vi "Laboratory_practice10.vi"() -> ()   [LabVIEW 2021]
panel:
  out "volts":dbl
  in  "Wait time(ms)":dbl
  in  "number of samples":i32=100
  in  "rate":dbl=5000.0
  out "Waveform Graph":dynamicdata(graph)
  in  "Traditional DAQ Channel":tag
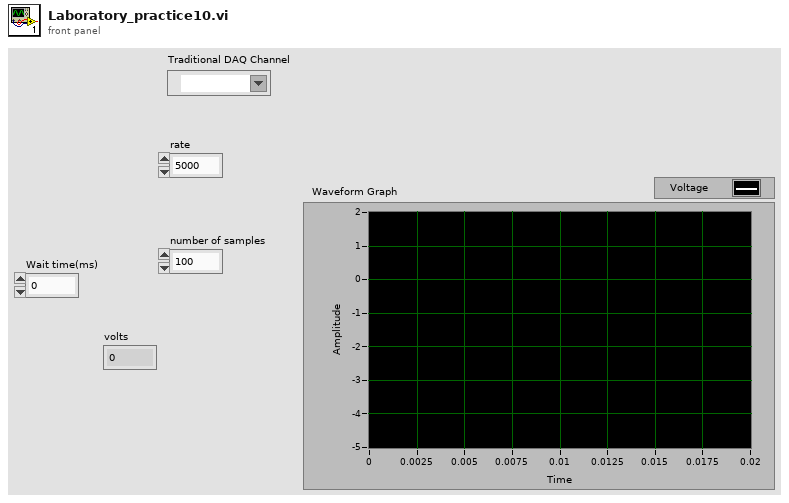
[diagram p1: front panel]
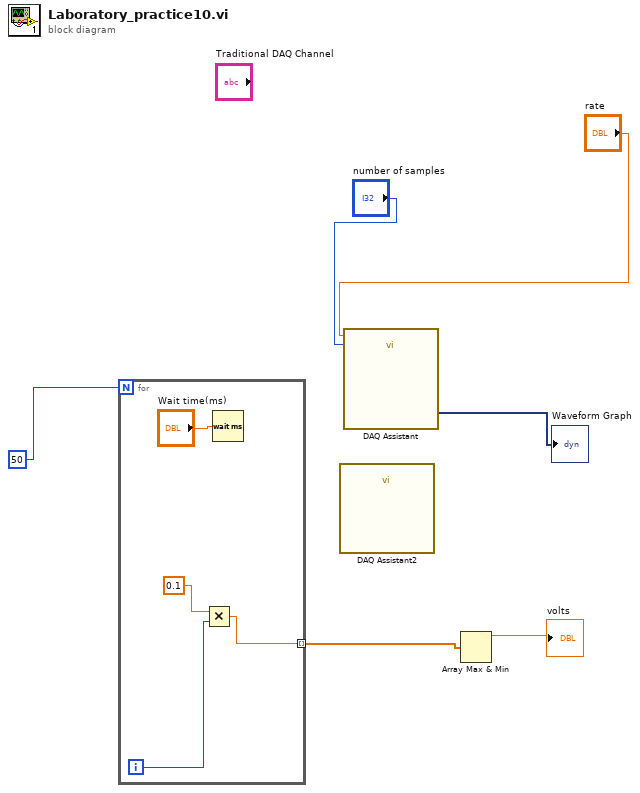
[diagram p0: block diagram]
diagram:
  n1 = for {
    N: 50 -> [_]
    tunnel: [w7] -> w2 mode=indexing
    i -> [w8]
    n2 = Multiply(x=0.1, y=w8) -> (x*y=w7:dbl)
    n3 = Wait (ms)(milliseconds to wait="Wait time(ms)") -> ()  [unwired: 1 out]
  }
  n4 = call "DAQ Assistant2"() -> ()  [unwired: 18 in, 2 out]
  n5 = call "DAQ Assistant"("rate"="rate", "number of samples"="number of samples") -> ("data"=→"Waveform Graph":dynamicdata)  [unwired: 15 in, 2 out]
  n6 = Array Max & Min(array=w2) -> (max value=→"volts":dbl)  [unwired: 3 out]
